vi "assemblies to tables.vi"(11 "assemblies":T1[](array[typedef])) -> (3 "Item Names":string[][](array[string]))   [LabVIEW 2013, in "EIP Tag API editor node.lvclass"]
uses:
  EIP Tag API editor node.lvclass
  <vilib>/NI/TBM Modules/Ethernet IP/configuration/assembly type.ctl
  <vilib>/NI/TBM Modules/Ethernet IP/configuration/assembly definition.ctl
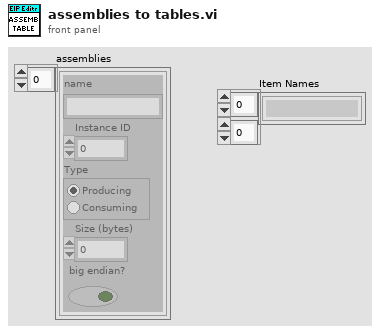
[diagram p1: front panel]
types:
  T1 = typedef "EthernetIP configuration.lvclass/assembly definition.ctl" = cluster{"name":string, "Instance ID":u32, "Type":T2, "Size (bytes)":u32, "big endian?":bool}
  T2 = typedef "EthernetIP configuration.lvclass/assembly type.ctl" = enum32{"Producing", "Consuming"}
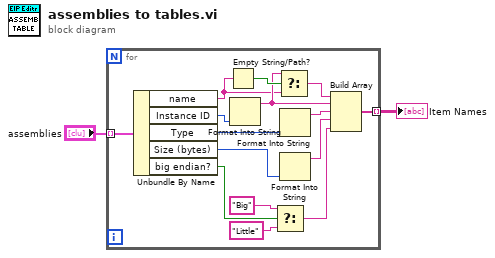
[diagram p0: block diagram]
diagram:
  n1 = for {
    tunnel: "assemblies" -> [w17] mode=indexing
    tunnel: [w11] -> w1 mode=indexing
    n2 = Unbundle By Name(w17) -> ("name"=w7:string, "Instance ID"=w14:u32, "Type"=w15:T2, "Size (bytes)"=w16:u32, "big endian?"=w4:bool)
    n3 = Empty String/Path?(string/path=w7) -> (empty?=w10:bool)
    n4 = Format Into String(w14) -> (resulting string=w8:string)  [unwired: 3 in, 1 out]
    n5 = Select(t="Big" ("resulting string"), s=w4, f="Little" ("resulting string")) -> (s? t:f=w3:string)
    n6 = Select(t=w8, s=w10, f=w7) -> (s? t:f=w9:string)
    n7 = Format Into String(w15) -> (resulting string=w13:string)  [unwired: 3 in, 1 out]
    n8 = Format Into String(w16) -> (resulting string=w12:string)  [unwired: 3 in, 1 out]
    n9 = Build Array(w9, w8, w13, w12, w3) -> (w11:string[])
  }
  "Item Names" <- w1
